vi "Diff_Drive_System_Globals.vi"() -> ()   [LabVIEW 2019]
panel:
  out "DrvSpeed READ Right":dbl format="%17.2f"
  out "DrvSpeed READ Left":dbl format="%17.2f"
  out "DrvFFLeft":dbl format="%17.2f"
  out "DrvFFRight":dbl format="%17.2f"
  out "DrvDmdAccelLeft":dbl format="%17.2f"
  out "DrvDmdAccelRight":dbl format="%17.2f"
  out "GyroRaw_DEG":dbl format="%17.2f"
  out "DrvDistCalcLeft":dbl format="%17.2f"
  out "DrvDistCalcRight":dbl format="%17.2f"
  out "DrvDistReadLeft":dbl format="%17.2f"
  out "DrvDistReadRight":dbl format="%17.2f"
  out "DrvSpeedLeft":dbl format="%17.2f"
  out "DrvSpeedRight":dbl format="%17.2f"
  out "DrvMotorOutLeft":dbl format="%17.2f"
  out "DrvMotorOutRight":dbl format="%17.2f"
  out "DrvSpeedDmdLeft":dbl format="%17.2f"
  out "DrvSpeedDmdRight":dbl format="%17.2f"
  out "DrvSpeedTargLeft":dbl format="%17.2f"
  out "DrvSpeedTargRight":dbl format="%17.2f"
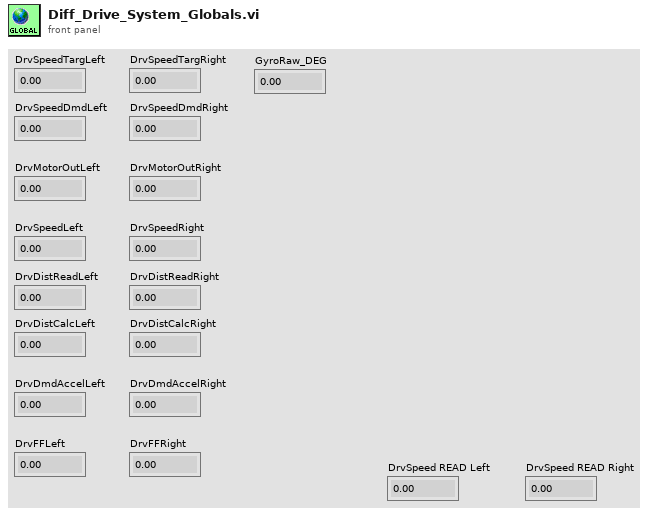
[diagram p1: front panel]
diagram:
